vi "CO Serial CAL & Data Recording & DECADEv3.3(serial_sim).vi"() -> ()   [LabVIEW 2014]
uses:
  <vilib>/Platform/TimedLoop/XDataNode/timing_clust.ctl
  <vilib>/Platform/TimedLoop/XDataNode/nitl_modes.ctl
  <vilib>/Platform/TimedLoop/XDataNode/wakeup.ctl
  C:/Program Files (x86)/National Instruments/LabVIEW 2014/examples/Data Communication/Network Streams/Simple Network Streams/support/Network Stream Command.ctl
  <vilib>/Utility/error.llb/whitespace.ctl
  <vilib>/Utility/tcp.llb/UDP Multicast Write-Only Open.vi
  <vilib>/Utility/tcp.llb/UDP Multicast Read-Only Open.vi
  <vilib>/Instr/_visa.llb/VISA Configure Serial Port (Instr).vi
  <vilib>/platform/TimedLoop/XDataNode/XDataNode.xnode
  <vilib>/Platform/TimedLoop/XDataNode/XDNodeRunTimeDep.lvlib
  <vilib>/NI_Real-Time Target Support.lvlib
panel:
  out "CO Vacuum":bool
  out "CO CAL":bool
  out "error out":errorcluster
  out "CO Vacuum?":i16
  out "Control data":i32[](array[numeric])
  out "Control data out":string
  in  "VISA resource name":refnum<visa-resource-name>="ASRL8::INSTR"
  out "Serial VISA error":errorcluster
  out "SEPTIC TCP Error Out":errorcluster
  out "TCP packet\nSend To SEPTIC":bool
  in  "msec to wait":u32=330 caption="mSec to Wait"
  in  "UDP Time Stamp\nOffset":u32=1
  out "Scan from String Error \nCounter from process loop":i32
  out "TCP Binary Packet":string
  in  "ue9LJ temp":u16
  out "FISH TCP Error Out":errorcluster
  out "TCP packet\nSend To FISH":bool
  out "UDP_In":string
  out "UDP_In_Error":errorcluster
  out "UDP_Out_Error Out":errorcluster
  out "Data Array":string[](array[string])
  out "UDP_Out Status":bool
  out "Data Process Status":bool
  out "Command In":string[](array[string])
  out "ERR Counter":i32
  out "UDP_Out":string
  out "UDP_Pack_num":u32
  in  "Flight Number":string
  in  "aux":string="0"
  in  "inlet_overq_mfm":string="0"
  in  "acs2653pc_hdd":string="0"
  in  "LabviewVIclient vn":string="0"
  in  "LabviewVIserver vn":string="0"
  out "cRIO CPU Total":string="0"
  in  "PTP Sync":string="0"
  out "OK RAW COUNTER":i32
  out "IN_CAL?":bool
  out "Redundent DATA":string
  out "Data String":string
  out "CO_Data_Buffer":string[](array[string])
  out "RAW DATA":string
  out "loop count":i32
  out "Number of Read error":i32
  out "Command In":string
  # "Pre-flight"
  # "CONC"
  # "SIG"
  # "SENS"
  # "ZERO"
  # "Lamp flow controller"
  # "Lamp temperature"
  # "Monochromater flow controller"
  # "Monochromater temperature"
  # "Monochromater pressure"
  # "Fluorescence cell pressure"
  # "Calibration gas pressure"
  # "Cell temperature"
  # "Calibration Concentration"
  # "ERROR number"
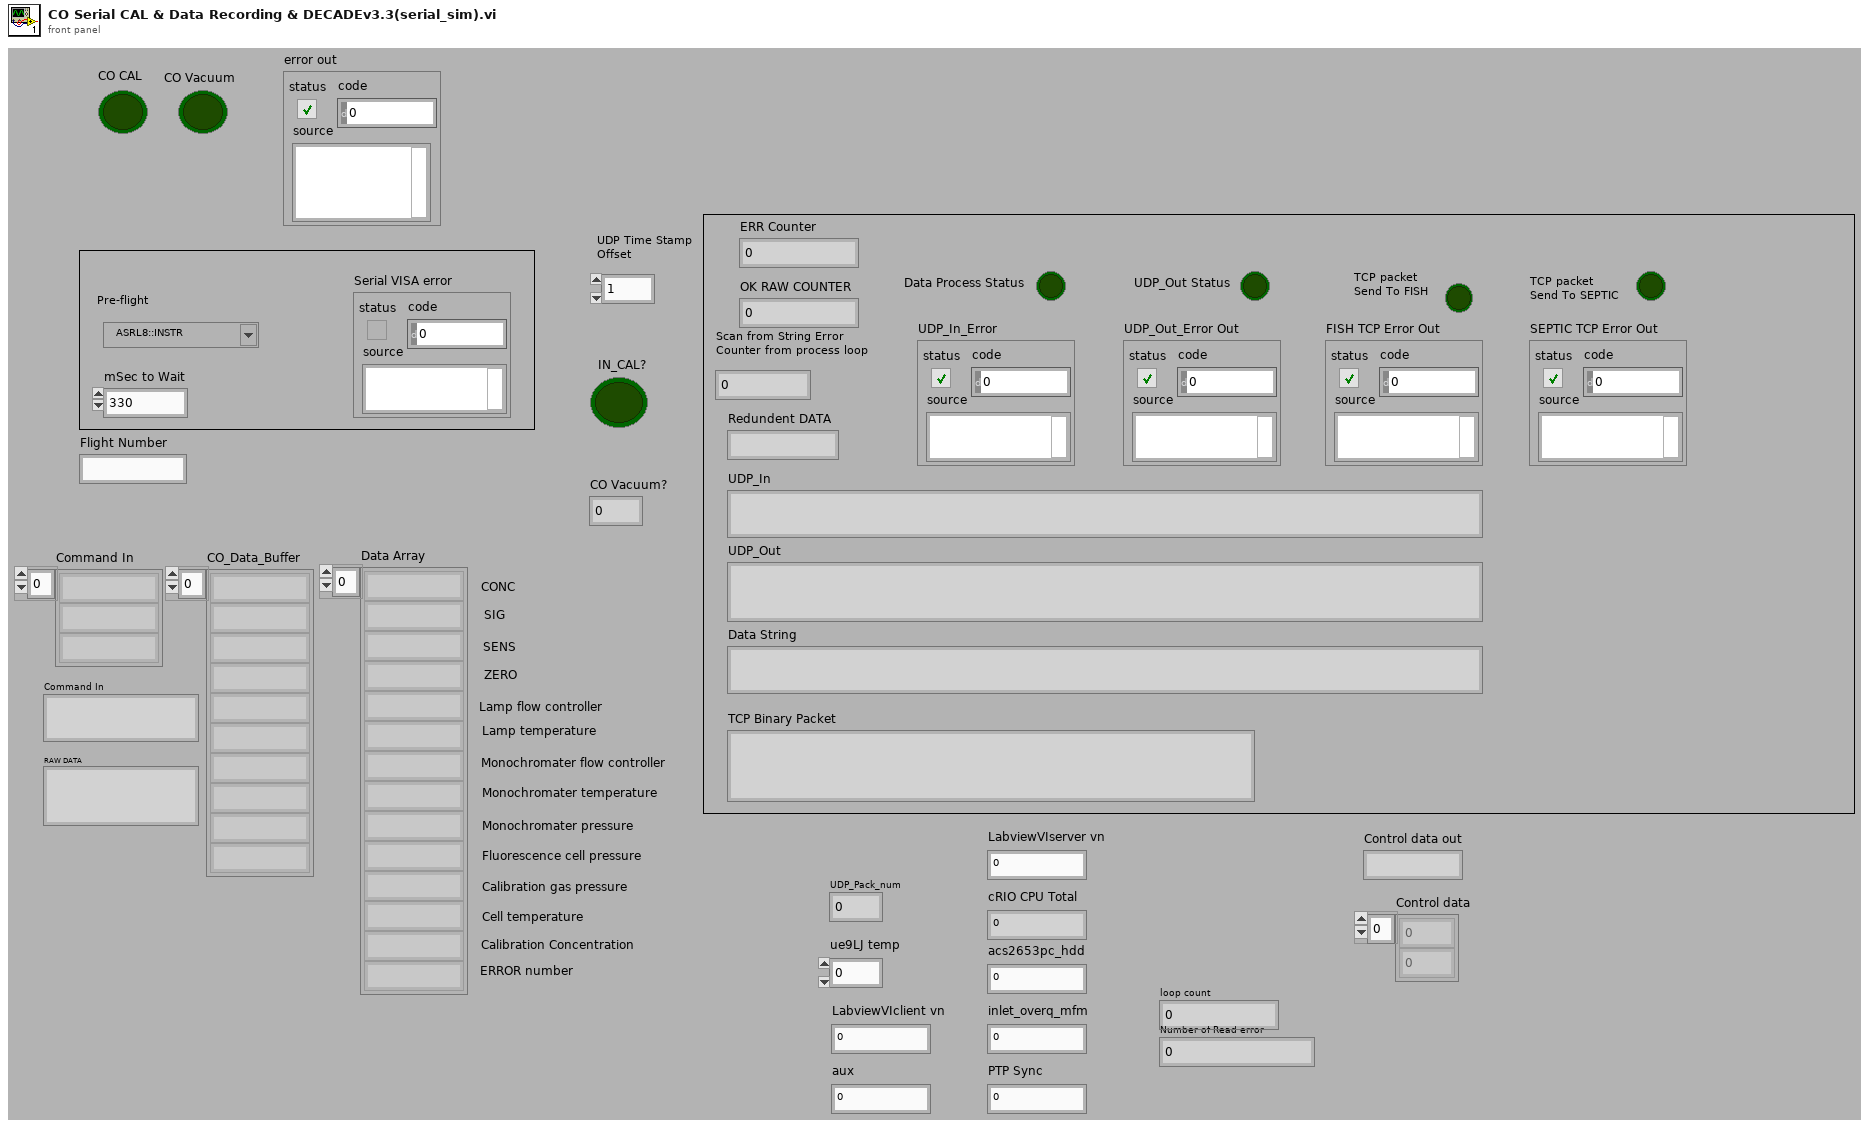
[diagram p1: front panel]
types:
  T1 = typedef "XDNodeRunTimeDep.lvlib/timing_clust.ctl" = cluster{"Expected End [f-1]":u64, "Actual End [f-1]":u64, "Finished Late? [f-1]":bool, "Expected End [i-1]":u64, "Actual End [i-1]":u64, "Finished Late? [i-1]":bool, "Expected Start [i]":u64, "Actual Start [i]":u64, "Expected Start [f]":u64, "Actual Start [f]":u64, "Source Name":string, "Structure Name":string, "Period":i64, "Deadline":i64, "Offset":i64, "Start":i64, "Priority":i32, "Timeout":i32, "Mode":T2, "Wakeup Reason":T3, "Error":errorcluster, "Source Type":string, "Secondary Source Type":string, "Global End Time":u64, "Global Start Time":u64, "Frame Duration":u64, "Iteration Duration":u64, "Assigned CPU":i32, "I/O Scan Engine Mode":u32}
  T2 = typedef "XDNodeRunTimeDep.lvlib/nitl_modes.ctl" = enum32{"No Change", "Process missed periods, maintain original phase", "Discard missed periods, maintain original phase", "Process missed periods, ignore original phase", "Discard missed periods, ignore original phase"}
  T3 = typedef "XDNodeRunTimeDep.lvlib/wakeup.ctl" = enum32{"Normal", "Aborted", "Asynchronous wakeup", "Timing source error", "Timed loop error", "Timeout"}
  T4 = typedef "Network Stream Command.ctl" = cluster{"Message":string, "Message Data":variant}
  T5 = typedef "NI_Real-Time Target Support.lvlib/RT CPU Load.ctl" = cluster{"Total (%)":dbl, "Time Critical (%)":dbl, "Timed Structures (%)":dbl, "High (%)":dbl, "Above Normal (%)":dbl, "Normal (%)":dbl, "Background (%)":dbl, "Idle (%)":dbl, "ISR (%)":dbl}
  T6 = typedef "whitespace.ctl" = u16
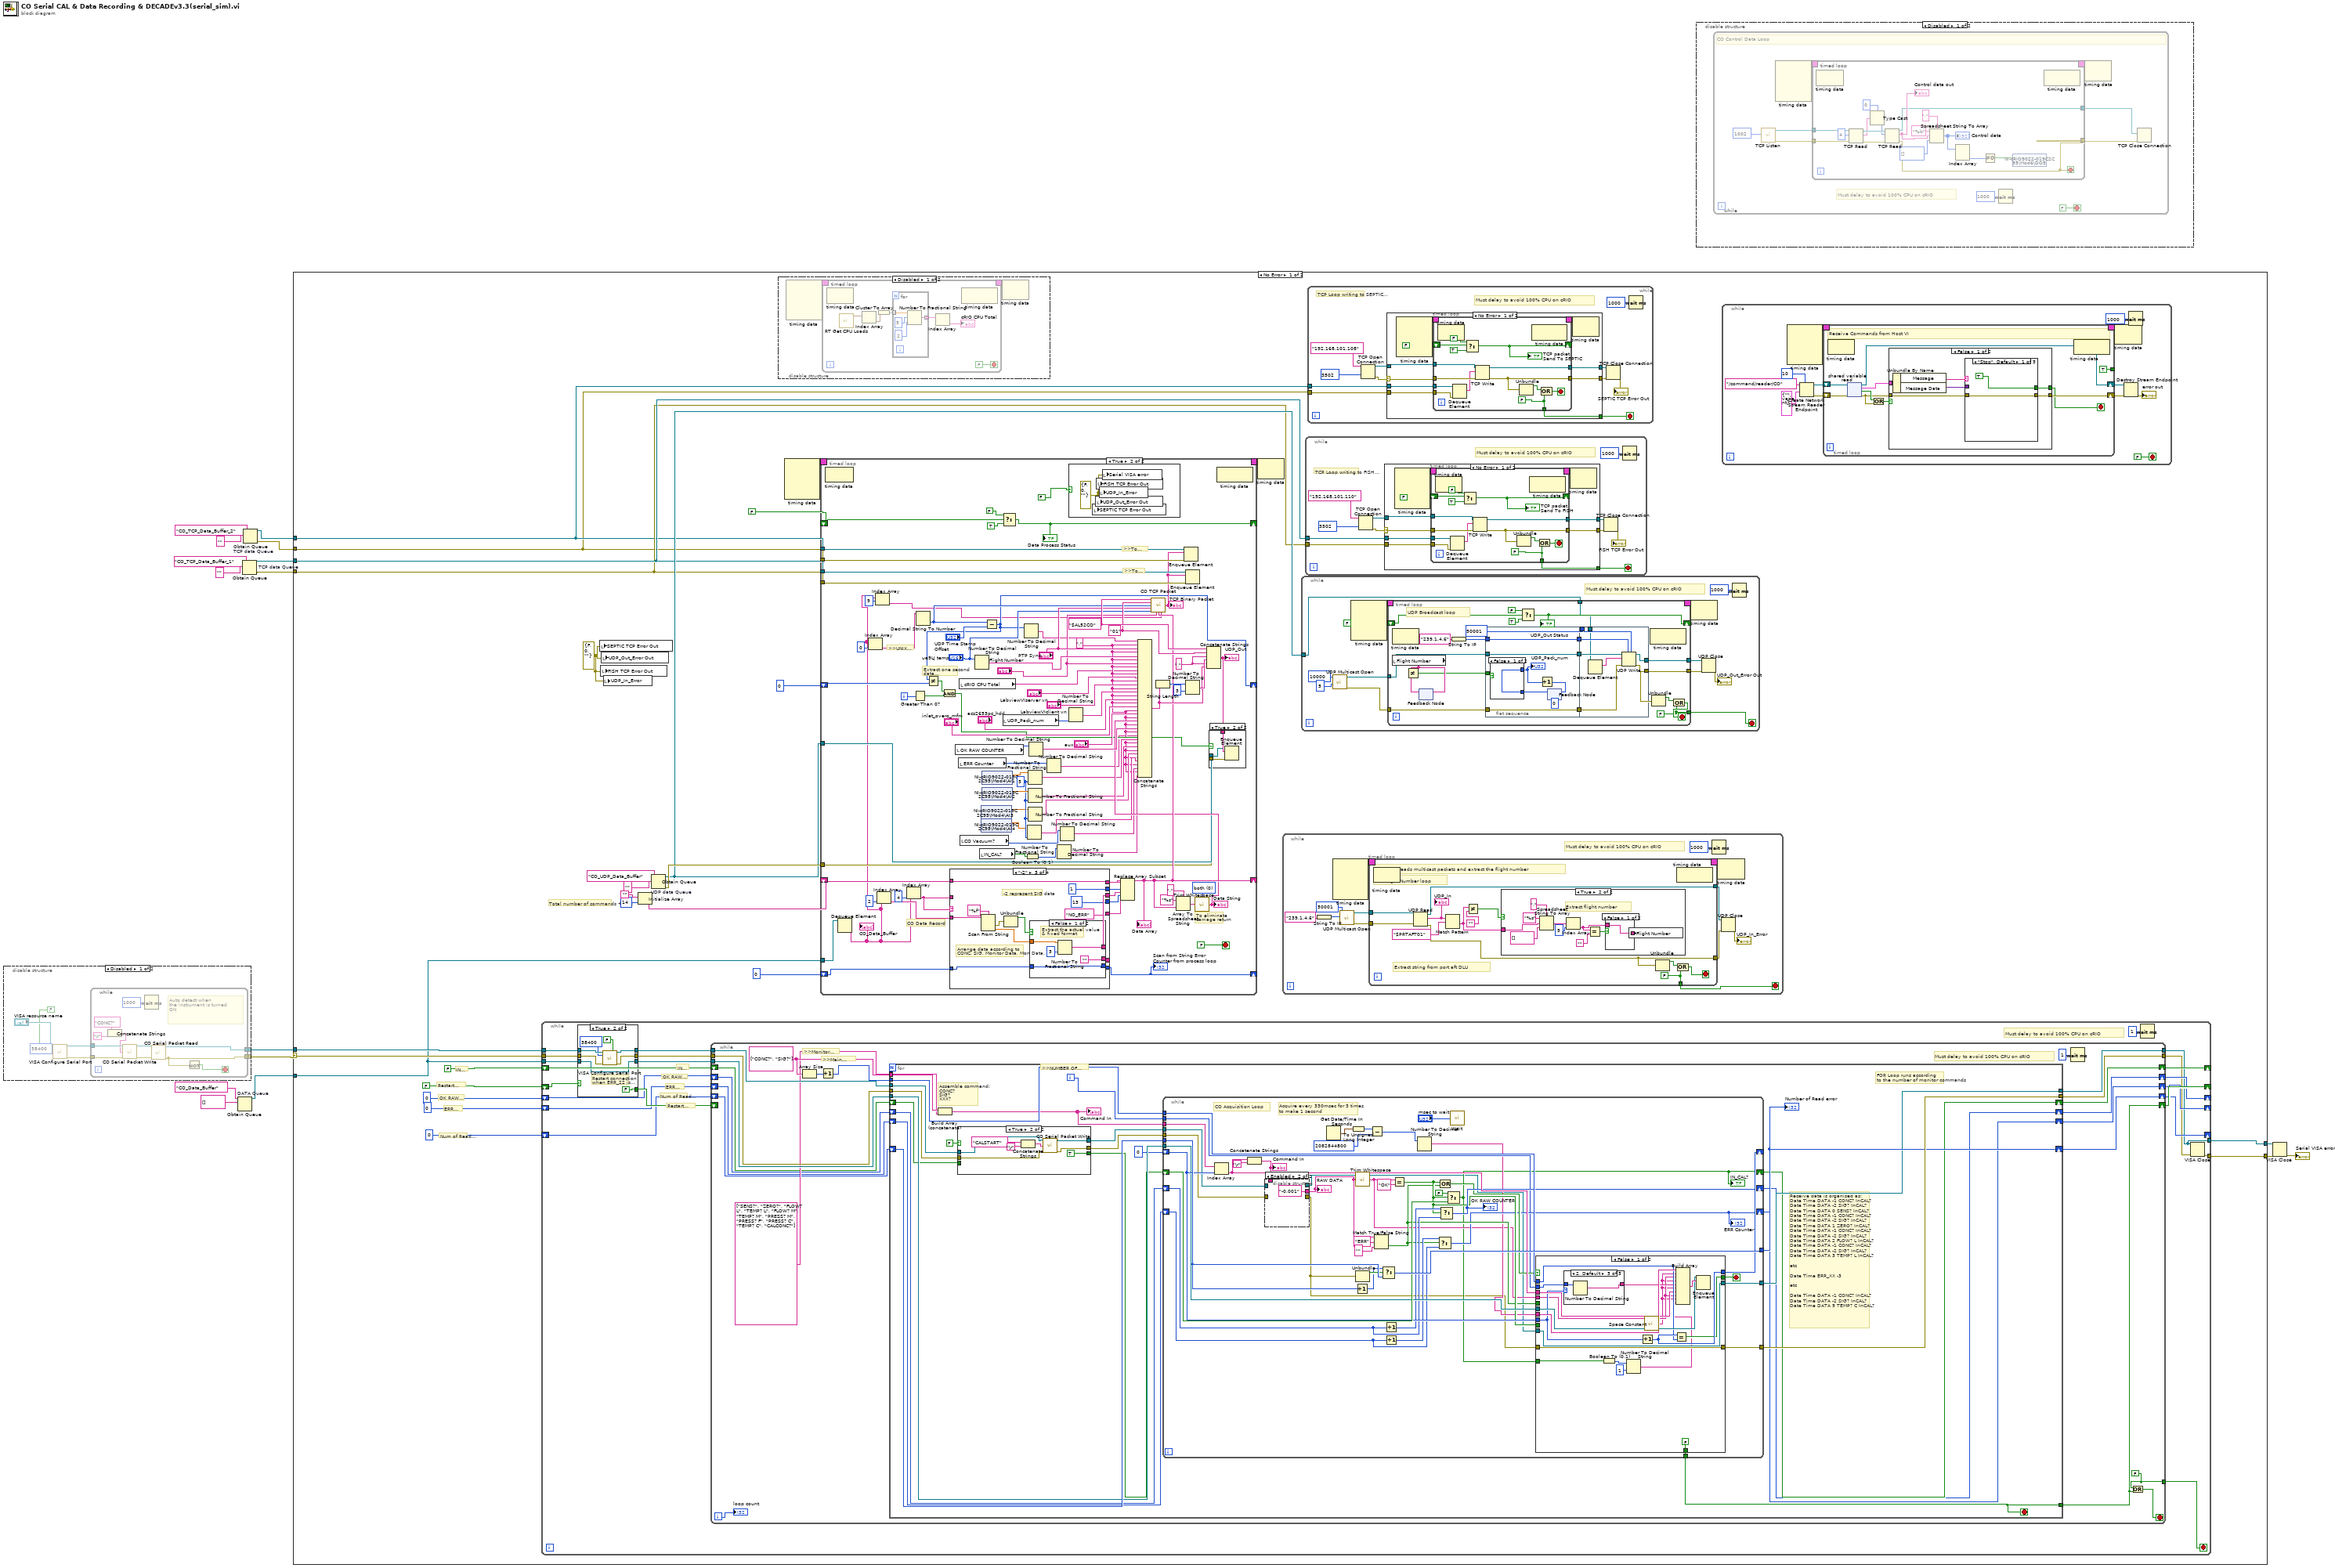
[diagram p0: block diagram]
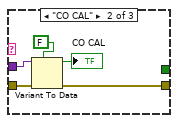
[diagram p5: hidden frame]
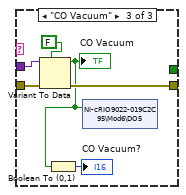
[diagram p6: hidden frame]
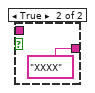
[diagram p9: hidden frame]
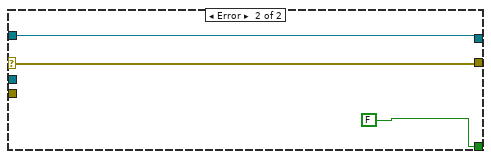
[diagram p10: hidden frame]
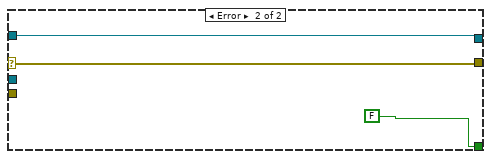
[diagram p11: hidden frame]
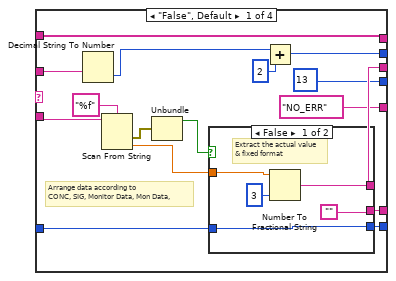
[diagram p14: hidden frame]
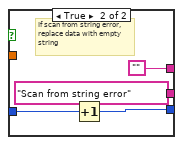
[diagram p15: hidden frame]
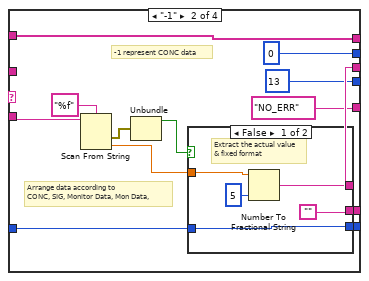
[diagram p16: hidden frame]
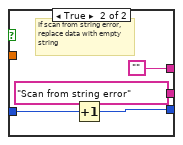
[diagram p17: hidden frame]
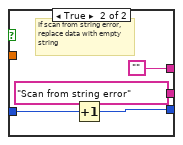
[diagram p18: hidden frame]
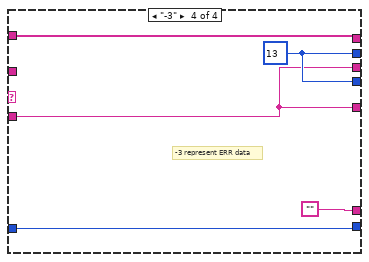
[diagram p19: hidden frame]
diagram:
  n1 = disable-structure shown="Disabled" {
    disable-tunnel: [w18 _] -> w6
    disable-tunnel: [w17 _] -> w5
    frame Disabled {
      n2 = call-poly "VISA Configure Serial Port"("VISA resource name"="VISA resource name", "Enable Termination\nChar (T)"=FALSE ("Enable Termination\nChar (T)"), "baud rate (9600)"=u32 38400) -> ("VISA resource name out"=w20:refnum<visa-resource-name>, "error out"=w19:errorcluster)  [unwired: 11 in]
      n3 = while {
        tunnel: w20 -> [w34]
        tunnel: w19 -> [w33]
        tunnel: [w27] -> w18
        tunnel: [w28] -> w17
        stop <- w32 stop-if-true
        # "Auto detect when\nthe instrument is turned \nON"
        n4 = Concatenate Strings("CONC?" ("Data in"), "\r") -> (w24:string)
        n5 = call "CO Serial Packet Write.vi"("VISA resource name In"=w34, "Data in"=w24, "error in (no error)"=w33) -> ("VISA resource name Out"=w30:refnum<visa-resource-name>, "error out"=w29:errorcluster)  [unwired: 11 in]
        n6 = Wait (ms)(milliseconds to wait=u32 1000) -> ()  [unwired: 1 out]
        n7 = call "CO Serial Packet Read.vi"("VISA resource In"=w30, "error in"=w29) -> ("VISA resource Out"=w27:refnum<visa-resource-name>, "error out"=w28:errorcluster)  [unwired: 11 in, 1 out]
        n8 = Not(x=w28) -> (.not. x?=w32:bool)
      }
    }
    frame Enabled {
    }
  }
  n9 = Obtain Queue "DATA Queue"(name (unnamed)="CO_Data_Buffer", element data type=string[] []) -> (queue out=w14:refnum<queue>)  [unwired: 3 in, 2 out]
  n10 = Obtain Queue "TCP data Queue"(name (unnamed)="CO_TCP_Data_Buffer_1", element data type="") -> (queue out=w13:refnum<queue>, error out=w12:errorcluster)  [unwired: 3 in, 1 out]
  n11 = Obtain Queue "TCP data Queue"(name (unnamed)="CO_TCP_Data_Buffer_2", element data type="") -> (queue out=w11:refnum<queue>, error out=w10:errorcluster)  [unwired: 3 in, 1 out]
  n12 = case shown="No Error" w5 {
    selector: w5 -> [w59 w668]
    tunnel: w6 -> [w60 w667]
    tunnel: [w61 w668] -> w8
    tunnel: [w37 w667] -> w7
    tunnel: w14 -> [w58 _]
    tunnel: w13 -> [w47 _]
    tunnel: w12 -> [w46 _]
    tunnel: w11 -> [w45 _]
    tunnel: w10 -> [w44 _]
    frame No Error {
      w43 = errorcluster {"status"=FALSE, "code"=0, "source"=""} ("UDP_Out_Error Out")
      # "Restart connection?"
      # "IN CAL?"
      # "OK RAW Counter"
      # "ERR Counter"
      # "Num of Read Error"
      # "Total number of commands + ERR"
      n13 = while {
        tunnel: [w419] -> w61
        tunnel: w60 -> [w436]
        tunnel: w59 -> [w435]
        tunnel: w58 -> [w433]
        shift-right: [w430] -> _
        shift-left: FALSE -> [w431]
        shift-right: [w426] -> _
        shift-left: 0 -> [w427]
        shift-right: [w423] -> _
        shift-left: 0 -> [w425]
        shift-right: [w422] -> _
        shift-left: 0 -> [w424]
        shift-right: [w420] -> _
        shift-left: FALSE ("IN_CAL?") -> [w421]
        tunnel: [w417] -> w37
        stop <- w429 stop-if-true
        # "Must delay to avoid 100% CPU on cRIO"
        # "Restart connection?"
        # "Num of Read Error"
        # "ERR Counter"
        # "IN CAL?"
        # "OK RAW Counter"
        n14 = case shown="True" w431 {
          selector: w431 -> [w438 _]
          tunnel: [w441 w446] -> w437
          tunnel: w436 -> [w441 w447]
          tunnel: [w440 w445] -> w434
          tunnel: w435 -> [w440 w444]
          tunnel: [w439 w449] -> w432
          tunnel: w433 -> [w439 w449]
          tunnel: [w438 FALSE] -> w428
          frame False {
          }
          frame True {
            # "Restart connection\nwhen ERR_22 is detected"
            n15 = call-poly "VISA Configure Serial Port"("VISA resource name"=w447, "Enable Termination\nChar (T)"=FALSE ("Enable Termination\nChar (T)"), "baud rate (9600)"=u32 38400, "error in (no error)"=w444) -> ("VISA resource name out"=w446:refnum<visa-resource-name>, "error out"=w445:errorcluster)  [unwired: 10 in]
          }
        }
        n16 = while {
          tunnel: [w471] -> w418
          tunnel: w437 -> [w470]
          tunnel: w434 -> [w469]
          tunnel: [w468] -> w417
          tunnel: w432 -> [w467]
          shift-right: [w458] -> w426
          shift-left: w427 -> [w462]
          shift-right: [w457] -> w423
          shift-left: w425 -> [w461]
          shift-right: [w456] -> w420
          shift-left: w421 -> [w460]
          shift-right: [w455] -> w422
          shift-left: w424 -> [w459]
          tunnel: [w451] -> w429
          shift-right: [w452] -> w430
          shift-left: w428 -> [_]
          i -> [w454]
          stop <- w453 stop-if-true
          w451 = FALSE
          w466 = string[] ["CONC?", "SIG?"]
          # "Must delay to avoid 100% CPU on cRIO"
          # ">>Main commands>>"
          # ">>Monitor Command>>"
          n17 = Array Size(array=w466) -> (size(s)=w463:i32)
          n18 = Increment(x=w463) -> (x+1=w465:i32)
          n19 = for {
            tunnel: w470 -> [w490]
            tunnel: w469 -> [w489]
            tunnel: [w495] -> w471
            shift-right: [w493] -> w455
            shift-left: w459 -> [w494]
            tunnel: [w492] -> w468
            tunnel: w467 -> [w491]
            tunnel: w465 -> [w485]
            shift-right: [w483] -> w456
            shift-left: w460 -> [w484]
            shift-right: [w481] -> w457
            shift-left: w461 -> [w482]
            shift-right: [w479] -> w458
            shift-left: w462 -> [w480]
            tunnel: string[] ["SENS?", "ZERO?", "FLOW? L", "TEMP? L", "FLOW? M", "TEMP? M", "PRESS? M", "PRESS? F", "PRESS? C", "TEMP? C", "CALCONC?"] -> [w476] mode=indexing
            tunnel: w466 -> [w477]
            tunnel: [w474] -> w452
            i -> [w475]
            stop <- w474 stop-if-true
            # "Receive data is organised as:\nDate Time DATA -1 CONC? InCAL?\nDate Time DATA -2 SIG? InCAL?\nDate Time DATA 0 SENS? InCAL?\nDate Time DATA -1 CONC? InCAL?\nDate Time DATA -2 SIG? InCAL?\nDate Time DATA 1 ZERO? InCAL?\nDate Time DATA -1 CONC? InCAL?\nDate Time DATA -2 SIG? InCAL?\nDate Time DATA 2 FLOW? L InCAL?\nDate Time DATA -1 CONC? InCAL?\nDate Time DATA -2 SIG? InCAL?\nDate Time DATA 3 TEMP? L InCAL?\n\netc\n\nDate Time ERR_XX -3\n\netc\n\nDate Time DATA -1 CONC? InCAL?\nDate Time DATA -2 SIG? InCAL?\nDate Time DATA 9 TEMP? C InCAL?"
            # "FOR Loop runs according\nto the number of monitor commands"
            # "Assemble command:\nCONC?\nSIG?\nXXX?"
            # ">>NUMBER OF COMMANDS>>"
            n20 = Build Array (concatenate)(w477, w476) -> (w478:string[])
            "Command In" <- w478
            n21 = case shown="True" FALSE {
              tunnel: w490 -> [w602 w604]
              tunnel: w489 -> [w601 w607]
              tunnel: [w602 w605] -> w488
              tunnel: [w601 w606] -> w487
              tunnel: [w600 TRUE ("IN_CAL?")] -> w486
              tunnel: w484 -> [w600 _]
              frame False {
              }
              frame True {
                n22 = Concatenate Strings("CALSTART" ("string"), "\r") -> (w603:string)
                n23 = call "CO Serial Packet Write.vi"("VISA resource name In"=w604, "Data in"=w603, "error in (no error)"=w607) -> ("VISA resource name Out"=w605:refnum<visa-resource-name>, "error out"=w606:errorcluster)  [unwired: 11 in]
              }
            }
            n24 = while {
              tunnel: w487 -> [w499]
              tunnel: [w527] -> w495
              tunnel: w494 -> [w539]
              tunnel: [w538] -> w493
              tunnel: w478 -> [w531]
              tunnel: [w528] -> w492
              tunnel: w491 -> [w526]
              tunnel: w488 -> [w501]
              shift-right: [w502] -> w483
              shift-left: w486 -> [w533]
              shift-right: [w530] -> _
              shift-left: 0 -> [w532]
              tunnel: w485 -> [w523]
              shift-right: [w520] -> w481
              shift-left: w482 -> [w521]
              shift-right: [w514] -> w479
              shift-left: w480 -> [w516]
              tunnel: w475 -> [w513]
              tunnel: [w507] -> w474
              stop <- w529 stop-if-true
              # "Acquire every 330msec for 3 times\nto make 1 second"
              # "CO Acquisition Loop"
              n25 = Index Array(array=w531, index=w532) -> (element=w525:string)
              n26 = Concatenate Strings(w525, "\r") -> (w500:string)
              "Command In" <- w500
              n27 = disable-structure shown="Enabled" {
                disable-tunnel: w501 -> [w547 _]
                disable-tunnel: w500 -> [w546 _]
                disable-tunnel: w499 -> [w545 _]
                disable-tunnel: [w542 _] -> w498
                disable-tunnel: [w541 _] -> w497
                disable-tunnel: [w540 "-0.001" ("RAW DATA")] -> w496
                frame Disabled {
                  n28 = call "CO Serial Packet Write.vi"("VISA resource name In"=w547, "Data in"=w546, "error in (no error)"=w545) -> ("VISA resource name Out"=w543:refnum<visa-resource-name>, "error out"=w544:errorcluster)  [unwired: 11 in]
                  n29 = call "CO Serial Packet Read.vi"("VISA resource In"=w543, "error in"=w544) -> ("VISA resource Out"=w542:refnum<visa-resource-name>, "Data Out"=w540:string, "error out"=w541:errorcluster)  [unwired: 11 in]
                }
                frame Enabled {
                }
              }
              "RAW DATA" <- w496
              n30 = Get Date/Time In Seconds() -> (seconds since 1Jan1904=w508:timestamp)
              n31 = To Unsigned Long Integer(number=w508) -> (unsigned 32bit integer=w512:u32)
              n32 = Increment(x=w539) -> (x+1=w535:i32)
              n33 = call <vilib>:"Trim Whitespace.vi"("string"=w496) -> ("trimmed string"=w506:string)  [unwired: 1 in]
              n34 = Unbundle(w497) -> ("status"=w536:bool)  [unwired: 2 out]
              n35 = Subtract(x=w512, y=u32 2082844800) -> (x-y=w503:u32)
              n36 = Match True/False String(2:"" ("false string"), 3:"ERR" ("true string"), 4:w496) -> (0:w515:bool)  [unwired: 1 out]
              n37 = Select(t=w535, s=w536, f=w539) -> (s? t:f=w538:i32)
              n38 = Increment(x=w521) -> (x+1=w522:i32)
              n39 = Increment(x=w516) -> (x+1=w517:i32)
              n40 = Equal?(x=w506, y="OK" ("string")) -> (x = y?=w518:bool)
              n41 = Number To Decimal String(number=w503) -> (decimal integer string=w510:string)  [unwired: 1 in]
              n42 = Select(t=w517, s=w515, f=w516) -> (s? t:f=w514:i32)
              "ERR Counter" <- w514
              n43 = Select(t=w522, s=w518, f=w521) -> (s? t:f=w520:i32)
              "OK RAW COUNTER" <- w520
              n44 = Compound Arithmetic op=OR(w518, w515) -> (w519:bool)
              n45 = Select(t=FALSE, s=w518, f=w533) -> (s? t:f=w502:bool)
              "IN_CAL?" <- w502
              n46 = call "Wait"("Count(mSec)"="msec to wait") -> ()  [unwired: 1 out]
              n47 = case shown="False" w519 {
                tunnel: w532 -> [w556 w584]
                tunnel: [w567 w584] -> w530
                tunnel: [w561 w574] -> w529
                tunnel: w498 -> [w566 w583]
                tunnel: w497 -> [w565 w582]
                tunnel: [w566 w581] -> w528
                tunnel: [w565 w580] -> w527
                tunnel: w526 -> [w563 w578]
                tunnel: w506 -> [w554 w576]
                tunnel: w525 -> [w557 _]
                tunnel: w510 -> [w562 w577]
                tunnel: w515 -> [_ w579]
                tunnel: w523 -> [w560 _]
                tunnel: w518 -> [_ w575]
                tunnel: w513 -> [w559 _]
                tunnel: [FALSE w572] -> w507
                tunnel: w502 -> [w553 _]
                frame False {
                  n48 = case shown="2, Default" w556 {
                    tunnel: w559 -> [_ _ w571]
                    tunnel: ["-1" "-2" w570] -> w558
                    frame 0 {
                      # "-1 represent CONC data"
                    }
                    frame 1 {
                      # "-2 represent SIG data"
                    }
                    frame 2, Default {
                      n49 = Number To Decimal String(number=w571) -> (decimal integer string=w570:string)  [unwired: 1 in]
                    }
                  }
                  n50 = Boolean To (0,1)(Boolean=w553) -> (0, 1=w552:i16)
                  n51 = Number To Decimal String(number=w552, width (-)=i16 1) -> (decimal integer string=w549:string)
                  n52 = Increment(x=w556) -> (x+1=w567:i32)
                  n53 = call <vilib>:"Space Constant.vi"() -> ("String"=w550:string)
                  n54 = Equal?(x=w567, y=w560) -> (x = y?=w561:bool)
                  n55 = Build Array(w562, w550, w554, w550, w558, w550, w557, w554, w550, w549) -> (w564:string[])
                  n56 = Enqueue Element(queue=w563, element=w564) -> ()  [unwired: 2 in, 3 out]
                }
                frame True {
                  # ">>REPEAT DATA REQUEST>>\nif OK or ERR"
                  n57 = case shown="True" w579 {
                    tunnel: w578 -> [_ w599]
                    tunnel: w577 -> [_ w597]
                    tunnel: w576 -> [_ w596]
                    tunnel: [FALSE TRUE] -> w572
                    frame False {
                    }
                    frame True {
                      # "-3 represent ERR data"
                      # "Send Error message\nthrough but repeat\ndata request"
                      n58 = call <vilib>:"Space Constant.vi"() -> ("String"=w595:string)
                      n59 = Build Array(w597, w595, w596, w595, "-3" ("element")) -> (w598:string[])
                      n60 = Enqueue Element(queue=w599, element=w598) -> ()  [unwired: 2 in, 3 out]
                    }
                  }
                  n61 = case shown="True" w575 {
                    tunnel: w583 -> [w585 w590]
                    tunnel: w582 -> [w586 w591]
                    tunnel: [w585 w589] -> w581
                    tunnel: [w586 w587] -> w580
                    frame False {
                    }
                    frame True {
                      # "Carry on reading packet\nif there is OK but\ndisregard the OK packet"
                      n62 = call "CO Serial Packet Read.vi"("VISA resource In"=w590, "error in"=w591) -> ("VISA resource Out"=w589:refnum<visa-resource-name>, "Data Out"=→"Redundent DATA":string, "error out"=w587:errorcluster)  [unwired: 11 in]
                    }
                  }
                  n63 = Or(x=w572, y=FALSE) -> (x .or. y?=w574:bool)
                }
              }
            }
            "Number of Read error" <- w493
          }
          n64 = Wait (ms)(milliseconds to wait=u32 1) -> ()  [unwired: 1 out]
          n65 = Or(x=w451, y=w452) -> (x .or. y?=w453:bool)
          "loop count" <- w454
        }
        n66 = Wait (ms)(milliseconds to wait=u32 1) -> ()  [unwired: 1 out]
        n67 = VISA Close(VISA resource name=w417, error in (no error)=w418) -> (error out=w419:errorcluster)
      }
      n68 = local write "SEPTIC TCP Error Out"(w43) -> ()
      n69 = local write "FISH TCP Error Out"(w43) -> ()
      n70 = local write "UDP_Out_Error Out"(w43) -> ()
      n71 = local write "UDP_In_Error"(w43) -> ()
      n72 = Initialize Array("", 14) -> (w55:string[])
      n73 = Obtain Queue "UDP data Queue"(name (unnamed)="CO_UDP_Data_Buffer", element data type="") -> (queue out=w50:refnum<queue>, error out=w51:errorcluster)  [unwired: 3 in, 1 out]
      n74 = disable-structure shown="Disabled" {
        frame Disabled {
          n75 = node-c288() -> (w63:T1)  [unwired: 4 in]
          n76 = timed-loop {
            timing: w63 -> [_]
            timing-out: [_] -> w62
            stop <- FALSE stop-if-true
            n77 = node-c288() -> ()  [unwired: 1 in, 1 out]
            n78 = call <vilib>:"RT Get CPU Loads.vi"() -> ("CPU loads"=w69:T5[])  [unwired: 10 in, 1 out]
            n79 = Index Array(array=w69) -> (element=w68:T5)  [unwired: 1 in]
            n80 = Cluster To Array(cluster=w68) -> (array=w67:dbl[])
            n81 = for {
              tunnel: w67 -> [w73] mode=indexing
              tunnel: [w70] -> w66 mode=indexing
              n82 = Number To Fractional String(number=w73, width (-)=i16 5, precision (6)=i16 2) -> (F-format string=w70:string)  [unwired: 1 in]
            }
            n83 = Index Array(array=w66) -> (element=→"cRIO CPU Total":string)  [unwired: 1 in]
            n84 = node-c288() -> ()  [unwired: 1 in, 1 out]
          }
          n85 = node-c288(w62) -> ()  [unwired: 1 out]
        }
        frame Enabled {
        }
      }
      n86 = node-c288() -> (w36:T1)  [unwired: 4 in]
      n87 = timed-loop {
        tunnel: w58 -> [w333]
        shift-right: [w295] -> _
        shift-left: w55 -> [w315]
        shift-right: [w302] -> _
        shift-left: FALSE -> [w305]
        tunnel: w47 -> [w294]
        tunnel: w46 -> [w293]
        tunnel: w50 -> [w290]
        tunnel: w51 -> [w289]
        shift-right: [w287] -> _
        shift-left: 0 -> [w288]
        shift-right: [w273] -> _
        shift-left: 0 -> [w281]
        tunnel: w45 -> [w279]
        tunnel: w44 -> [w278]
        timing: w36 -> [_]
        timing-out: [_] -> w35
        i -> [w284]
        stop <- FALSE stop-if-true
        w264 = i16 3 ("precision (6)")
        w307 = T6 0 items=["both", "start of string", "end of string"] ("location (both)")
        w253 = ","
        w300 = "01"
        w318 = ","
        w301 = "$AL52CO"
        # ">>To SEPTIC>>"
        # ">>To FISH>>"
        # "Extract one second data\nfor UDP sending"
        # ">>UNIX TIME>>"
        # "To eliminate\ncarriage return"
        # "CO Data Record"
        n88 = node-c288() -> ()  [unwired: 1 in, 1 out]
        n89 = Dequeue Element(queue=w333) -> (element=w269:string[])  [unwired: 2 in, 3 out]
        "CO_Data_Buffer" <- w269
        n90 = Index Array(array=w269, index=0) -> (element=w282:string)
        n91 = Index Array(array=w269, index=9) -> (element=w268:string)
        n92 = Index Array(array=w269, index=2) -> (element=w313:string)
        n93 = Index Array(array=w269, index=4) -> (element=w314:string)
        n94 = Greater Than 0?(x=w284) -> (x > 0?=w283:bool)
        n95 = Decimal String To Number(string=w282) -> (number=w276:i32)  [unwired: 2 in, 1 out]
        n96 = case shown="\"-2\"" w314 {
          tunnel: w314 -> [w354 _ _ _]
          tunnel: w315 -> [w355 w377 w399 w413]
          tunnel: w313 -> [w346 w371 w393 w409]
          tunnel: [w355 w377 w399 w413] -> w312
          tunnel: [w352 0 ("index") 1 ("index") w410] -> w311
          tunnel: [w345 w367 w389 w409] -> w310
          tunnel: [w344 w368 w390 ""] -> _
          tunnel: w288 -> [w343 w370 w392 w411]
          tunnel: [w342 w369 w391 w411] -> w287
          tunnel: [13 ("index") 13 ("index") 13 ("index") w410] -> w272
          tunnel: ["NO_ERR" "NO_ERR" "NO_ERR" w409] -> w271
          frame "False", Default {
            # "Arrange data according to\nCONC, SIG, Monitor Data, Mon Data,"
            n97 = Decimal String To Number(string=w354) -> (number=w351:i32)  [unwired: 2 in, 1 out]
            n98 = Scan From String(format string="%f", input string=w346) -> (error out=w348:errorcluster, output 1=w349:dbl)  [unwired: 3 in, 2 out]
            n99 = Unbundle(w348) -> ("status"=w347:bool)  [unwired: 2 out]
            n100 = case shown="False" w347 {
              tunnel: [w360 ""] -> w345
              tunnel: w349 -> [w359 _]
              tunnel: w343 -> [w358 w363]
              tunnel: [w358 w362] -> w342
              tunnel: ["" "Scan from string error"] -> w344
              frame False {
                # "Extract the actual value\n& fixed format"
                n101 = Number To Fractional String(number=w359, precision (6)=i16 3) -> (F-format string=w360:string)  [unwired: 2 in]
              }
              frame True {
                # "If scan from string error,\nreplace data with empty\nstring"
                n102 = Increment(x=w363) -> (x+1=w362:i32)
              }
            }
            n103 = Add(x=w351, y=2) -> (x+y=w352:i32)
          }
          frame "-1" {
            # "Arrange data according to\nCONC, SIG, Monitor Data, Mon Data,"
            # "-1 represent CONC data"
            n104 = Scan From String(format string="%f", input string=w371) -> (error out=w373:errorcluster, output 1=w374:dbl)  [unwired: 3 in, 2 out]
            n105 = Unbundle(w373) -> ("status"=w372:bool)  [unwired: 2 out]
            n106 = case shown="False" w372 {
              tunnel: [w382 ""] -> w367
              tunnel: w374 -> [w381 _]
              tunnel: w370 -> [w380 w385]
              tunnel: [w380 w384] -> w369
              tunnel: ["" "Scan from string error"] -> w368
              frame False {
                # "Extract the actual value\n& fixed format"
                n107 = Number To Fractional String(number=w381, precision (6)=i16 5) -> (F-format string=w382:string)  [unwired: 2 in]
              }
              frame True {
                # "If scan from string error,\nreplace data with empty\nstring"
                n108 = Increment(x=w385) -> (x+1=w384:i32)
              }
            }
          }
          frame "-2" {
            # "Arrange data according to\nCONC, SIG, Monitor Data, Mon Data,"
            # "-2 represent SIG data"
            n109 = Scan From String(format string="%f", input string=w393) -> (error out=w395:errorcluster, output 1=w396:dbl)  [unwired: 3 in, 2 out]
            n110 = Unbundle(w395) -> ("status"=w394:bool)  [unwired: 2 out]
            n111 = case shown="False" w394 {
              tunnel: [w404 ""] -> w389
              tunnel: w396 -> [w403 _]
              tunnel: w392 -> [w402 w407]
              tunnel: [w402 w406] -> w391
              tunnel: ["" "Scan from string error"] -> w390
              frame False {
                # "Extract the actual value\n& fixed format"
                n112 = Number To Fractional String(number=w403, precision (6)=i16 3) -> (F-format string=w404:string)  [unwired: 2 in]
              }
              frame True {
                # "If scan from string error,\nreplace data with empty\nstring"
                n113 = Increment(x=w407) -> (x+1=w406:i32)
              }
            }
          }
          frame "-3" {
            w410 = 13 ("index")
            # "-3 represent ERR data"
          }
        }
        "Scan from String Error \nCounter from process loop" <- w287
        n114 = local read "OK RAW COUNTER"() -> (w316:i32)
        n115 = local read "ERR Counter"() -> (w251:i32)
        n116 = local read "cRIO CPU Total"() -> (w249:string)
        n117 = local read "CO Vacuum?"() -> (w255:i16)
        n118 = Number To Decimal String(number="ue9LJ temp") -> (decimal integer string=w298:string)  [unwired: 1 in]
        n119 = local read "IN_CAL?"() -> (w263:bool)
        n120 = shared-variable "NI-cRIO9022-019C2C95\\Mod4\\AI3"() -> (w261:dbl)  [unwired: 1 in, 1 out]
        n121 = shared-variable "NI-cRIO9022-019C2C95\\Mod4\\AI4"() -> (w260:dbl)  [unwired: 1 in, 1 out]
        n122 = shared-variable "NI-cRIO9022-019C2C95\\Mod4\\AI1"() -> (w266:dbl)  [unwired: 1 in, 1 out]
        n123 = shared-variable "NI-cRIO9022-019C2C95\\Mod4\\AI2"() -> (w265:dbl)  [unwired: 1 in, 1 out]
        n124 = Subtract(x=w276, y="UDP Time Stamp\nOffset") -> (x-y=w273:u32)
        n125 = Not Equal?(x=w273, y=w281) -> (x != y?=w285:bool)
        n126 = Compound Arithmetic op=AND(w285, w283) -> (w280:bool)
        n127 = Select(t=FALSE, s=w305, f=TRUE) -> (s? t:f=w302:bool)
        "Data Process Status" <- w302
        n128 = local read "UDP_Pack_num"() -> (w327:u32)
        n129 = Number To Decimal String(number=w273) -> (decimal integer string=w274:string)  [unwired: 1 in]
        n130 = Boolean To (0,1)(Boolean=w263) -> (0, 1=w262:i16)
        n131 = Number To Fractional String(number=w260, precision (6)=w264) -> (F-format string=w256:string)  [unwired: 2 in]
        n132 = Number To Fractional String(number=w266, precision (6)=w264) -> (F-format string=w259:string)  [unwired: 2 in]
        n133 = Number To Fractional String(number=w265, precision (6)=w264) -> (F-format string=w258:string)  [unwired: 2 in]
        n134 = Number To Fractional String(number=w261, precision (6)=w264) -> (F-format string=w257:string)  [unwired: 2 in]
        n135 = Number To Decimal String(number=w316) -> (decimal integer string=w322:string)  [unwired: 1 in]
        n136 = Number To Decimal String(number=w251) -> (decimal integer string=w250:string)  [unwired: 1 in]
        n137 = Number To Decimal String(number=w262) -> (decimal integer string=w252:string)  [unwired: 1 in]
        n138 = Number To Decimal String(number=w255) -> (decimal integer string=w254:string)  [unwired: 1 in]
        n139 = Number To Decimal String(number=w327) -> (decimal integer string=w326:string)  [unwired: 1 in]
        n140 = case shown="True" FALSE {
          frame False {
          }
          frame True {
            w336 = errorcluster {"status"=FALSE, "code"=0, "source"=""} ("UDP_Out_Error Out")
            n141 = local write "SEPTIC TCP Error Out"(w336) -> ()
            n142 = local write "UDP_Out_Error Out"(w336) -> ()
            n143 = local write "FISH TCP Error Out"(w336) -> ()
            n144 = local write "UDP_In_Error"(w336) -> ()
            n145 = local write "Serial VISA error"(w336) -> ()
          }
        }
        n146 = Replace Array Subset(array=w312, new element #1=w310, index #1=w311, new element #2=w271, index #2=w272) -> (w295:string[])
        "Data Array" <- w295
        n147 = call "CO TCP Packet.vi"("ID"=w301, "Version"=w300, "utc_time"=w276, "PTP Sync"="PTP Sync", "ue9LJ temp"="ue9LJ temp", "Flight Number"="Flight Number", "Data Array"=w295, "In_CAL?"=w268) -> ("TCP Binary Packet"=w277:string)  [unwired: 7 in]
        "TCP Binary Packet" <- w277
        n148 = Array To Spreadsheet String(delimiter (Tab)=",", array=w295, 3:"%s" ("format string")) -> (spreadsheet string=w306:string)
        n149 = Enqueue Element(queue=w279, element=w277, error in (no error)=w278) -> ()  [unwired: 1 in, 3 out]
        n150 = Enqueue Element(queue=w294, element=w277, error in (no error)=w293) -> ()  [unwired: 1 in, 3 out]
        n151 = call <vilib>:"Trim Whitespace.vi"("string"=w306, "location (both)"=w307) -> ("trimmed string"=w292:string)
        "Data String" <- w292
        n152 = Concatenate Strings(w274, w253, "PTP Sync", w253, w298, w253, "Flight Number", w253, w249, w253, "LabviewVIserver vn", w253, "LabviewVIclient vn", w253, w326, w253, "acs2653pc_hdd", w253, "inlet_overq_mfm", w253, "aux", w253, w292, w253, w322, w253, w250, w259, w253, w258, w253, w257, w253, w256, w253, w254, w253, w252) -> (w317:string)
        n153 = String Length(string=w317) -> (length=w321:i32)
        n154 = Number To Decimal String(number=w321, width (-)=i16 3) -> (decimal integer string=w319:string)
        n155 = Concatenate Strings(w301, w300, w318, w319, w318, w317) -> (w291:string)
        "UDP_Out" <- w291
        n156 = case shown="True" w280 {
          tunnel: w291 -> [_ w339]
          tunnel: w290 -> [_ w338]
          tunnel: w289 -> [_ w337]
          frame False {
          }
          frame True {
            n157 = Enqueue Element(queue=w338, element=w339, error in (no error)=w337) -> ()  [unwired: 1 in, 3 out]
          }
        }
        n158 = node-c288() -> ()  [unwired: 1 in, 1 out]
      }
      n159 = node-c288(w35) -> ()  [unwired: 1 out]
      n160 = while {
        stop <- w126 stop-if-true
        # "Must delay to avoid 100% CPU on cRIO"
        n161 = String To IP(1:"239.1.4.6" ("name")) -> (0:w134:u32)
        n162 = node-c288() -> (w136:T1)  [unwired: 4 in]
        n163 = call-poly <vilib>:"UDP Multicast Open.vi"("multicast addr"=w134, "port"=u16 50001) -> ("error out"=w130:errorcluster, "connection ID"=w131:refnum<k16>)  [unwired: 7 in, 1 out]
        n164 = timed-loop {
          tunnel: w131 -> [w148]
          tunnel: w130 -> [w147]
          timing: w136 -> [_]
          timing-out: [_] -> w135
          tunnel: [w141] -> w128
          tunnel: [w139] -> w127
          tunnel: [w137] -> w126
          stop <- w138 stop-if-true
          w137 = FALSE
          # "Extract string from port aft DLU"
          # "Get Flight Number loop"
          # "This loop reads multicast packets and extract the flight number"
          n165 = node-c288() -> ()  [unwired: 1 in, 1 out]
          n166 = UDP Read(connection ID=w148, 8:w147) -> (data out=w146:string, error out=w139:errorcluster, 3:w141:refnum<k16>)  [unwired: 2 in, 2 out]
          "UDP_In" <- w146
          n167 = Match Pattern(string=w146, regular expression="$PRTAFT01") -> (after substring=w142:string)  [unwired: 1 in, 3 out]
          n168 = Not Equal?(x=w142, y="") -> (x != y?=w143:bool)
          n169 = case shown="True" w143 {
            tunnel: w142 -> [_ w155]
            frame False {
            }
            frame True {
              # "Extract flight number"
              n170 = Spreadsheet String To Array(delimiter (Tab)=",", format string="%s", spreadsheet string=w155, array type (2D Dbl)=string[] []) -> (array=w157:string[])
              n171 = Index Array(array=w157, index=5) -> (element=w151:string)
              n172 = Equal?(x=w151, y="") -> (x = y?=w154:bool)
              n173 = case shown="False" w154 {
                tunnel: [w161 "XXXX"] -> w152
                tunnel: w151 -> [w161 _]
                frame False {
                }
                frame True {
                }
              }
              n174 = local write "Flight Number"(w152) -> ()
            }
          }
          n175 = Unbundle(w139) -> ("status"=w140:bool)  [unwired: 2 out]
          n176 = node-c288() -> ()  [unwired: 1 in, 1 out]
          n177 = Compound Arithmetic op=OR(w140, w137) -> (w138:bool)
        }
        n178 = Wait (ms)(milliseconds to wait=u32 1000) -> ()  [unwired: 1 out]
        n179 = node-c288(w135) -> ()  [unwired: 1 out]
        n180 = UDP Close(connection ID=w128, 8:w127) -> (error out=→"UDP_In_Error":errorcluster)  [unwired: 1 out]
      }
      n181 = while {
        tunnel: w50 -> [w612]
        stop <- w613 stop-if-true
        # "Must delay to avoid 100% CPU on cRIO"
        n182 = call-poly <vilib>:"UDP Multicast Open.vi"("time-to-live (1)"=u16 5, "port"=u16 10000) -> ("error out"=w620:errorcluster, "connection ID"=w621:refnum<k16>)  [unwired: 8 in]
        n183 = node-c288() -> (w623:T1)  [unwired: 4 in]
        n184 = timed-loop {
          tunnel: w621 -> [w643]
          tunnel: w620 -> [w642]
          timing: w623 -> [_]
          timing-out: [_] -> w622
          shift-right: [w630] -> _
          shift-left: FALSE -> [w633]
          tunnel: [w629] -> w615
          tunnel: [w627] -> w614
          tunnel: [w625] -> w613
          tunnel: w612 -> [w624]
          stop <- w626 stop-if-true
          w625 = FALSE
          # "UDP Broadcast loop"
          n185 = node-c288() -> ()  [unwired: 1 in, 1 out]
          n186 = local read "Flight Number"() -> (w636:string)
          n187 = feedback-in #1(w636) -> ()
          n188 = feedback #1() -> (w635:string)  [unwired: 1 in]
          n189 = Not Equal?(x=w636, y=w635) -> (x != y?=w634:bool)
          n190 = String To IP(1:"239.1.4.6" ("name")) -> (0:w640:u32)
          n191 = flat-sequence {
            tunnel: w640 -> [w650]
            tunnel: w642 -> [w651]
            tunnel: w643 -> [w652]
            tunnel: [w652] -> w639
            tunnel: [w651] -> w638
            tunnel: [w650] -> w637
            tunnel: w634 -> [w649]
            tunnel: u16 50001 ("port or service name") -> [w662]
            tunnel: w639 -> [w661]
            tunnel: w638 -> [w660]
            tunnel: w637 -> [w659]
            tunnel: [w658] -> w629
            tunnel: [w657] -> w627
            tunnel: w624 -> [w655]
            frame #0 {
              n192 = feedback #2(u32 0) -> (w646:u32)
              n193 = case shown="False" w649 {
                tunnel: w646 -> [w653 _]
                tunnel: [w653 u32 0] -> w645
                frame False {
                }
                frame True {
                }
              }
              "UDP_Pack_num" <- w645
              n194 = Increment(x=w645) -> (x+1=w647:u32)
              n195 = feedback-in #2(w647) -> ()
            }
            frame #1 {
              n196 = Dequeue Element(queue=w655) -> (element=w656:string)  [unwired: 2 in, 3 out]
              n197 = UDP Write(address=w659, port or service name=w662, connection ID=w661, data in=w656, 8:w660) -> (error out=w657:errorcluster, 3:w658:refnum<k16>)  [unwired: 1 in]
            }
          }
          n198 = Select(t=FALSE, s=w633, f=TRUE) -> (s? t:f=w630:bool)
          "UDP_Out Status" <- w630
          n199 = node-c288() -> ()  [unwired: 1 in, 1 out]
          n200 = Unbundle(w627) -> ("status"=w628:bool)  [unwired: 2 out]
          n201 = Compound Arithmetic op=OR(w628, w625) -> (w626:bool)
        }
        n202 = node-c288(w622) -> ()  [unwired: 1 out]
        n203 = UDP Close(connection ID=w615, 8:w614) -> (error out=→"UDP_Out_Error Out":errorcluster)  [unwired: 1 out]
        n204 = Wait (ms)(milliseconds to wait=u32 1000) -> ()  [unwired: 1 out]
      }
      n205 = while {
        tunnel: w47 -> [w209]
        tunnel: w46 -> [w208]
        stop <- w212 stop-if-true
        # "Must delay to avoid 100% CPU on cRIO"
        # "TCP Loop writing to FISH Tank"
        n206 = TCP Open Connection(address="192.168.101.110", remote port or service name=u16 3502) -> (connection ID=w215:refnum<k5>, error out=w210:errorcluster)  [unwired: 3 in]
        n207 = case shown="No Error" w210 {
          selector: w210 -> [w220 w247]
          tunnel: w215 -> [w225 w248]
          tunnel: [w224 w248] -> w214
          tunnel: [w223 w247] -> w213
          tunnel: [w222 FALSE] -> w212
          tunnel: w209 -> [w219 _]
          tunnel: w208 -> [w218 _]
          frame No Error {
            n208 = node-c288() -> (w227:T1)  [unwired: 4 in]
            n209 = timed-loop {
              tunnel: w225 -> [w241]
              tunnel: w220 -> [w240]
              tunnel: [w239] -> w224
              tunnel: [w238] -> w223
              tunnel: [w228] -> w222
              shift-right: [w232] -> _
              shift-left: FALSE -> [w235]
              timing: w227 -> [_]
              timing-out: [_] -> w226
              tunnel: w219 -> [w231]
              tunnel: w218 -> [w230]
              stop <- w236 stop-if-true
              w228 = FALSE
              n210 = node-c288() -> ()  [unwired: 1 in, 1 out]
              n211 = Dequeue Element(queue=w231, error in (no error)=w230) -> (element=w229:string)  [unwired: 1 in, 3 out]
              n212 = Select(t=FALSE, s=w235, f=TRUE) -> (s? t:f=w232:bool)
              "TCP packet\nSend To FISH" <- w232
              n213 = TCP Write(connection ID=w241, data in=w229, error in (no error)=w240) -> (connection ID out=w239:refnum<k5>, error out=w238:errorcluster)  [unwired: 1 in, 1 out]
              n214 = Unbundle(w238) -> ("status"=w237:bool)  [unwired: 2 out]
              n215 = node-c288() -> ()  [unwired: 1 in, 1 out]
              n216 = Compound Arithmetic op=OR(w237, w228) -> (w236:bool)
            }
            n217 = node-c288(w226) -> ()  [unwired: 1 out]
          }
          frame Error {
          }
        }
        n218 = TCP Close Connection(connection ID=w214, error in (no error)=w213) -> (error out=→"FISH TCP Error Out":errorcluster)  [unwired: 1 in, 1 out]
        n219 = Wait (ms)(milliseconds to wait=u32 1000) -> ()  [unwired: 1 out]
      }
      n220 = while {
        tunnel: w45 -> [w167]
        tunnel: w44 -> [w166]
        stop <- w170 stop-if-true
        # "Must delay to avoid 100% CPU on cRIO"
        # "TCP Loop writing to SEPTIC Tank"
        n221 = TCP Open Connection(address="192.168.101.108", remote port or service name=u16 3502) -> (connection ID=w173:refnum<k5>, error out=w168:errorcluster)  [unwired: 3 in]
        n222 = case shown="No Error" w168 {
          selector: w168 -> [w178 w205]
          tunnel: w173 -> [w183 w206]
          tunnel: [w182 w206] -> w172
          tunnel: [w181 w205] -> w171
          tunnel: [w180 FALSE] -> w170
          tunnel: w167 -> [w177 _]
          tunnel: w166 -> [w176 _]
          frame No Error {
            n223 = node-c288() -> (w185:T1)  [unwired: 4 in]
            n224 = timed-loop {
              tunnel: w183 -> [w199]
              tunnel: w178 -> [w198]
              tunnel: [w197] -> w182
              tunnel: [w196] -> w181
              tunnel: [w186] -> w180
              shift-right: [w190] -> _
              shift-left: FALSE -> [w193]
              timing: w185 -> [_]
              timing-out: [_] -> w184
              tunnel: w177 -> [w189]
              tunnel: w176 -> [w188]
              stop <- w194 stop-if-true
              w186 = FALSE
              n225 = node-c288() -> ()  [unwired: 1 in, 1 out]
              n226 = Dequeue Element(queue=w189, error in (no error)=w188) -> (element=w187:string)  [unwired: 1 in, 3 out]
              n227 = Select(t=FALSE, s=w193, f=TRUE) -> (s? t:f=w190:bool)
              "TCP packet\nSend To SEPTIC" <- w190
              n228 = TCP Write(connection ID=w199, data in=w187, error in (no error)=w198) -> (connection ID out=w197:refnum<k5>, error out=w196:errorcluster)  [unwired: 1 in, 1 out]
              n229 = Unbundle(w196) -> ("status"=w195:bool)  [unwired: 2 out]
              n230 = node-c288() -> ()  [unwired: 1 in, 1 out]
              n231 = Compound Arithmetic op=OR(w195, w186) -> (w194:bool)
            }
            n232 = node-c288(w184) -> ()  [unwired: 1 out]
          }
          frame Error {
          }
        }
        n233 = TCP Close Connection(connection ID=w172, error in (no error)=w171) -> (error out=→"SEPTIC TCP Error Out":errorcluster)  [unwired: 1 in, 1 out]
        n234 = Wait (ms)(milliseconds to wait=u32 1000) -> ()  [unwired: 1 out]
      }
      n235 = while {
        stop <- FALSE stop-if-true
        n236 = node-c288() -> (w79:T1)  [unwired: 4 in]
        n237 = Create Network Stream Reader Endpoint(7:10 ("reader buffer size"), 9:T4 {"Message"="", "Message Data"=variant} ("Message Cluster"), 11:"/command/reader/CO" ("reader url")) -> (0:w85:errorcluster, 3:w86:refnum<k21>)  [unwired: 4 in]
        n238 = timed-loop "Host->Target Command Reader" {
          shift-right: [w96] -> w83
          shift-left: w85 -> [w99]
          shift-right: [w97] -> w82
          shift-left: w86 -> [w98]
          tunnel: [TRUE] -> _
          timing: w79 -> [_]
          timing-out: [_] -> w78
          stop <- w90 stop-if-true
          # "Receive Commands from Host VI"
          n239 = node-c288() -> ()  [unwired: 1 in, 1 out]
          n240 = shared-variable-read(w98, w99) -> (w97:refnum<k21>, w92:errorcluster, w94:bool, w95:T4)  [unwired: 1 in]
          n241 = Or(x=w94, y=w92) -> (x .or. y?=w93:bool)
          n242 = case shown="False" w93 {
            selector: w93 -> [_ w121]
            tunnel: w92 -> [w107 w122]
            tunnel: [w106 w122] -> w96
            tunnel: w95 -> [w104 _]
            tunnel: [w105 w121] -> w90
            frame False {
              n243 = Unbundle By Name(w104) -> ("Message"=w103:string, "Message Data"=w102:variant)
              n244 = case shown="\"Stop\", Default" w103 {
                tunnel: w107 -> [w109 w114 w120]
                tunnel: [w109 w113 w119] -> w106
                tunnel: w102 -> [_ w112 w118]
                tunnel: [TRUE _ _] -> w105
                frame "Stop", Default {
                }
                frame "CO CAL" {
                  n245 = Variant To Data(error in=w114, type=FALSE, Variant=w112) -> (data=→"CO CAL":bool, error out=w113:errorcluster)
                }
                frame "CO Vacuum" {
                  n246 = Variant To Data(error in=w120, type=FALSE, Variant=w118) -> (data=w115:bool, error out=w119:errorcluster)
                  "CO Vacuum" <- w115
                  n247 = Boolean To (0,1)(Boolean=w115) -> (0, 1=→"CO Vacuum?":i16)
                  n248 = shared-variable "NI-cRIO9022-019C2C95\\Mod6\\DO5"(w115) -> ()  [unwired: 1 in, 1 out]
                }
              }
            }
            frame True {
            }
          }
          n249 = node-c288() -> ()  [unwired: 1 in, 1 out]
        }
        n250 = node-c288(w78) -> ()  [unwired: 1 out]
        n251 = Destroy Stream Endpoint(8:w83, 11:w82) -> (0:→"error out":errorcluster)
        n252 = Wait (ms)(milliseconds to wait=u32 1000) -> ()  [unwired: 1 out]
      }
    }
    frame Error {
    }
  }
  n253 = disable-structure shown="Disabled" {
    frame Disabled {
      n254 = while {
        stop <- FALSE stop-if-true
        # "Must delay to avoid 100% CPU on cRIO"
        # "CO Control Data Loop"
        n255 = call <vilib>:"TCP Listen.vi"("port"=u16 1002) -> ("error out"=w673:errorcluster, "connection ID"=w674:refnum<k5>)  [unwired: 6 in, 3 out]
        n256 = node-c288() -> (w677:T1)  [unwired: 4 in]
        n257 = timed-loop {
          timing: w677 -> [_]
          timing-out: [_] -> w676
          tunnel: w674 -> [w694]
          tunnel: w673 -> [w693]
          tunnel: [w683] -> w672
          tunnel: [w682] -> w671
          stop <- w682 stop-if-true
          n258 = node-c288() -> ()  [unwired: 1 in, 1 out]
          n259 = TCP Read(connection ID=w694, bytes to read=4, error in (no error)=w693) -> (connection ID out=w691:refnum<k5>, data out=w688:string, error out=w690:errorcluster)  [unwired: 2 in]
          n260 = Type Cast(type=0, x=w688) -> (*(type *) &x=w687:i32)
          n261 = TCP Read(connection ID=w691, bytes to read=w687, error in (no error)=w690) -> (connection ID out=w683:refnum<k5>, data out=w684:string, error out=w682:errorcluster)  [unwired: 2 in]
          "Control data out" <- w684
          n262 = Spreadsheet String To Array(delimiter (Tab)=",", format string="%b", spreadsheet string=w684, array type (2D Dbl)=i32[] []) -> (array=w681:i32[])
          "Control data" <- w681
          n263 = Index Array(array=w681) -> (element #2=w679:i32)  [unwired: 2 in, 1 out]
          n264 = Not Equal To 0?(x=w679) -> (x != 0?=w678:bool)
          n265 = shared-variable "NI-cRIO9022-019C2C95\\Mod6\\DO5"(w678) -> ()  [unwired: 1 in, 1 out]
          n266 = node-c288() -> ()  [unwired: 1 in, 1 out]
        }
        n267 = Wait (ms)(milliseconds to wait=u32 1000) -> ()  [unwired: 1 out]
        n268 = node-c288(w676) -> ()  [unwired: 1 out]
        n269 = TCP Close Connection(connection ID=w672, error in (no error)=w671) -> ()  [unwired: 1 in, 2 out]
      }
    }
    frame Enabled {
    }
  }
  n270 = VISA Close(VISA resource name=w7, error in (no error)=w8) -> (error out=→"Serial VISA error":errorcluster)
